vi "Read Controllers.vi"   [LabVIEW 2014]
uses:
  Begin/Global RefNums.vi
  <vilib>/Rock Robotics/WPI/Joystick/WPI_JoystickGetSetRefNum.vi
  Begin/Global Variables.vi
  <vilib>/Rock Robotics/Network Tables/SD Write Number.vi
types:
  T1 = typedef "WPI_JoystickDevRef.ctl" = cluster{"Device":T2}
  T2 = typedef "WPI_JoystickDeviceEnum.ctl" = enum16{"USB 0", "USB 1", "USB 2", "USB 3", "USB 4", "USB 5"}
  T3 = cluster{"Axes[0]":dbl, "Axes[1]":dbl, "Axes[2]":dbl, "Axes[3]":dbl, "Axes[4]":dbl, "Axes[5]":dbl, "Axes[6]":dbl, "Axes[7]":dbl, "Axes[8]":dbl}
  T4 = cluster{"Buttons[0]":bool, "Buttons[1]":bool, "Buttons[2]":bool, "Buttons[3]":bool, "Buttons[4]":bool, "Buttons[5]":bool, "Buttons[6]":bool, "Buttons[7]":bool, "Buttons[8]":bool}
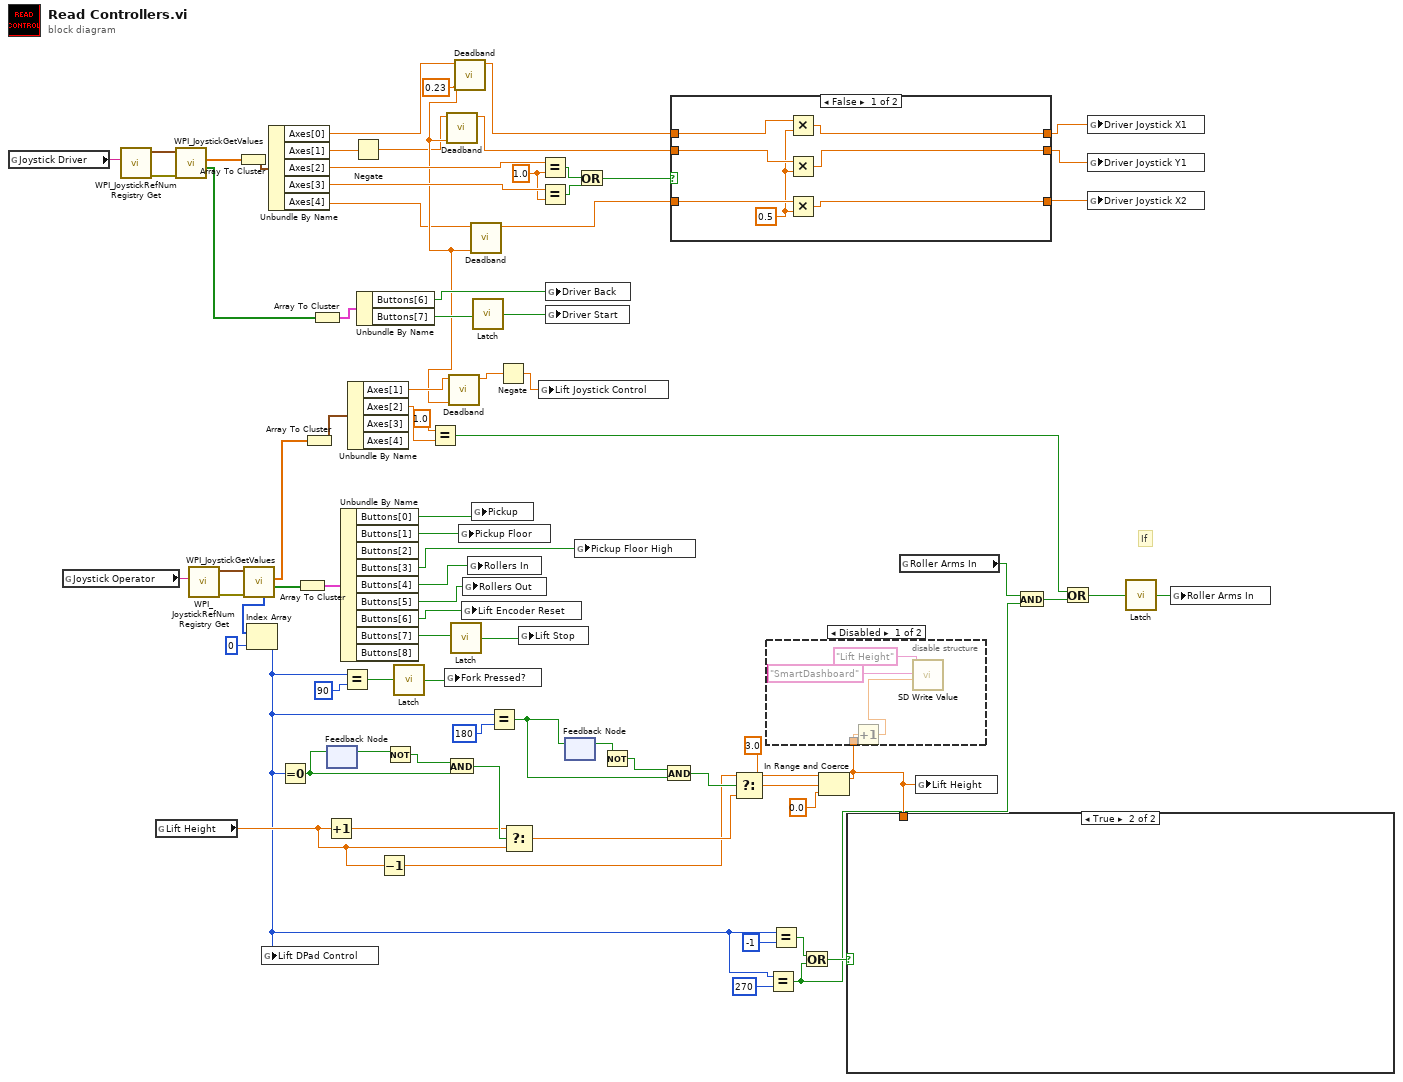
[diagram p0: block diagram]
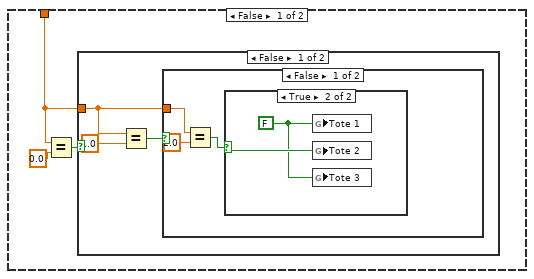
[diagram p2: hidden frame]
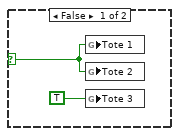
[diagram p3: hidden frame]
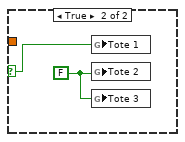
[diagram p4: hidden frame]
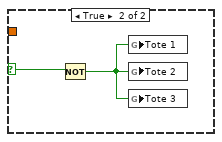
[diagram p5: hidden frame]
diagram:
  w22 = 0.23 ("Value to Deadband (default of 0.1)")
  w64 = 1.0 ("y")
  # "If"
  n1 = global read "Global RefNums.vi" "Joystick Driver"() -> (w80:string)
  n2 = global read "Global RefNums.vi" "Joystick Operator"() -> (w75:string)
  n3 = call <vilib>:"WPI_JoystickRefNum Registry Get.vi"("refnum name"=w80) -> ("error out"=w78:errorcluster, "JoystickDevRef"=w79:T1)  [unwired: 9 in]
  n4 = global read "Global Variables.vi" "Lift Height"() -> (w38:dbl)
  n5 = call <vilib>:"WPI_JoystickGetValues.vi"("error in (no error)"=w78, "JoystickDevRef"=w79) -> ("Buttons"=w63:bool[], "Axes"=w74:dbl[])  [unwired: 5 in, 3 out]
  n6 = call <vilib>:"WPI_JoystickRefNum Registry Get.vi"("refnum name"=w75) -> ("error out"=w77:errorcluster, "JoystickDevRef"=w76:T1)  [unwired: 9 in]
  n7 = Array To Cluster(array=w74) -> (cluster=w73:T3)
  n8 = call <vilib>:"WPI_JoystickGetValues.vi"("error in (no error)"=w77, "JoystickDevRef"=w76) -> ("Buttons"=w57:bool[], "Axes"=w29:dbl[], "POVs"=w51:i16[])  [unwired: 5 in, 2 out]
  n9 = Index Array(array=w51, index=0) -> (element=w11:i16)
  n10 = global write "Global Variables.vi" "Lift DPad Control"(w11) -> ()
  n11 = Unbundle By Name(w73) -> ("Axes[0]"=w58:dbl, "Axes[1]"=w13:dbl, "Axes[2]"=w69:dbl, "Axes[3]"=w65:dbl, "Axes[4]"=w14:dbl)
  n12 = Equal To 0?(x=w11) -> (x = 0?=w47:bool)
  n13 = Array To Cluster(array=w57) -> (cluster=w56:T4)
  n14 = Array To Cluster(array=w29) -> (cluster=w28:T3)
  n15 = Array To Cluster(array=w63) -> (cluster=w62:T4)
  n16 = Increment(x=w38) -> (x+1=w45:dbl)
  n17 = feedback-in #1(w47) -> ()
  n18 = feedback #1() -> (w49:bool)  [unwired: 1 in]
  n19 = Unbundle By Name(w56) -> ("Buttons[0]"=w55:bool, "Buttons[1]"=w54:bool, "Buttons[3]"=w15:bool, "Buttons[4]"=w26:bool, "Buttons[5]"=w25:bool, "Buttons[6]"=w24:bool, "Buttons[7]"=w53:bool)  [unwired: 2 out]
  n20 = Equal?(x=w11, y=i16 90) -> (x = y?=w9:bool)
  n21 = Unbundle By Name(w28) -> ("Axes[1]"=w23:dbl, "Axes[2]"=w16:dbl)  [unwired: 2 out]
  n22 = Negate(x=w13) -> (-x=w12:dbl)
  n23 = Unbundle By Name(w62) -> ("Buttons[6]"=w31:bool, "Buttons[7]"=w33:bool)
  n24 = Decrement(x=w38) -> (x-1=w37:dbl)
  n25 = Not(x=w49) -> (.not. x?=w48:bool)
  n26 = call "Latch.vi"("Input"=w9) -> ("Output"=w8:bool)
  n27 = Equal?(x=1.0, y=w16) -> (x = y?=w4:bool)
  n28 = global write "Global Variables.vi" "Fork Pressed?"(w8) -> ()
  n29 = call "Deadband.vi"("Value to Deadband (default of 0.1)"=w22, "Value"=w12) -> ("Deadbanded Value"=w60:dbl)  [unwired: 9 in]
  n30 = And(x=w48, y=w47) -> (x .and. y?=w46:bool)
  n31 = call "Deadband.vi"("Value to Deadband (default of 0.1)"=w22, "Value"=w23) -> ("Deadbanded Value"=w20:dbl)  [unwired: 9 in]
  n32 = call "Latch.vi"("Input"=w53) -> ("Output"=w52:bool)
  n33 = call "Deadband.vi"("Value to Deadband (default of 0.1)"=w22, "Value"=w58) -> ("Deadbanded Value"=w61:dbl)  [unwired: 9 in]
  n34 = global write "Global Variables.vi" "Pickup Floor"(w54) -> ()
  n35 = global write "Global Variables.vi" "Lift Encoder Reset"(w24) -> ()
  n36 = global write "Global Variables.vi" "Rollers Out"(w25) -> ()
  n37 = global write "Global Variables.vi" "Rollers In"(w26) -> ()
  n38 = call "Deadband.vi"("Value to Deadband (default of 0.1)"=w22, "Value"=w14) -> ("Deadbanded Value"=w59:dbl)  [unwired: 9 in]
  n39 = global write "Global Variables.vi" "Pickup"(w55) -> ()
  n40 = call "Latch.vi"("Input"=w33) -> ("Output"=w32:bool)
  n41 = Equal?(x=w11, y=i16 180) -> (x = y?=w43:bool)
  n42 = Negate(x=w20) -> (-x=w19:dbl)
  n43 = Select(t=w45, s=w46, f=w38) -> (s? t:f=w39:dbl)
  n44 = global write "Global Variables.vi" "Lift Stop"(w52) -> ()
  n45 = global write "Global Variables.vi" "Lift Joystick Control"(w19) -> ()
  n46 = Equal?(x=w69, y=w64) -> (x = y?=w67:bool)
  n47 = Equal?(x=w65, y=w64) -> (x = y?=w66:bool)
  n48 = global write "Global Variables.vi" "Driver Back"(w31) -> ()
  n49 = global write "Global Variables.vi" "Driver Start"(w32) -> ()
  n50 = feedback #2() -> (w42:bool)  [unwired: 1 in]
  n51 = feedback-in #2(w43) -> ()
  n52 = global write "Global Variables.vi" "Pickup Floor High"(w15) -> ()
  n53 = Or(x=w67, y=w66) -> (x .or. y?=w68:bool)
  n54 = Not(x=w42) -> (.not. x?=w41:bool)
  n55 = And(x=w41, y=w43) -> (x .and. y?=w40:bool)
  n56 = case shown="False" w68 {
    tunnel: w61 -> [w87 w88]
    tunnel: w60 -> [w86 w89]
    tunnel: w59 -> [w85 w90]
    tunnel: [w81 w90] -> w71
    tunnel: [w82 w89] -> w70
    tunnel: [w83 w88] -> w72
    frame False {
      w84 = 0.5 ("y")
      n57 = Multiply(x=w87, y=w84) -> (x*y=w83:dbl)
      n58 = Multiply(x=w86, y=w84) -> (x*y=w82:dbl)
      n59 = Multiply(x=w85, y=w84) -> (x*y=w81:dbl)
    }
    frame True {
    }
  }
  n60 = Select(t=w37, s=w40, f=w39) -> (s? t:f=w34:dbl)
  n61 = Equal?(x=w11, y=i16 270) -> (x = y?=w5:bool)
  n62 = Equal?(x=w11, y=i16 -1) -> (x = y?=w18:bool)
  n63 = Or(x=w18, y=w5) -> (x .or. y?=w7:bool)
  n64 = In Range and Coerce(upper limit=3.0, x=w34, lower limit=0.0) -> (coerced(x)=w30:dbl)  [unwired: 1 out]
  n65 = disable-structure shown="Disabled" {
    disable-tunnel: w30 -> [w92 _]
    frame Disabled {
      n66 = Increment(x=w92) -> (x+1=w91:dbl)
      n67 = call-poly <vilib>:"SD Write Value.vi"("Numeric"=w91, "Table Prefix"="SmartDashboard", "Name"="Lift Height") -> ()  [unwired: 7 in, 2 out]
    }
    frame Enabled {
    }
  }
  n68 = case shown="True" w7 {
    tunnel: w30 -> [w97 _]
    frame False {
      n69 = Equal?(x=w97, y=0.0) -> (x = y?=w96:bool)
      n70 = case shown="False" w96 {
        selector: w96 -> [_ w111]
        tunnel: w97 -> [w98 _]
        frame False {
          n71 = Equal?(x=w98, y=1.0) -> (x = y?=w99:bool)
          n72 = case shown="False" w99 {
            selector: w99 -> [_ w108]
            tunnel: w98 -> [w103 _]
            frame False {
              n73 = Equal?(x=w103, y=2.0) -> (x = y?=w101:bool)
              n74 = case shown="True" w101 {
                selector: w101 -> [w104 w107]
                frame False {
                  n75 = global write "Global Variables.vi" "Tote 1"(w104) -> ()
                  n76 = global write "Global Variables.vi" "Tote 2"(w104) -> ()
                  n77 = global write "Global Variables.vi" "Tote 3"(TRUE ("Tote 2")) -> ()
                }
                frame True {
                  w106 = FALSE ("Tote 0")
                  n78 = global write "Global Variables.vi" "Tote 1"(w106) -> ()
                  n79 = global write "Global Variables.vi" "Tote 2"(w107) -> ()
                  n80 = global write "Global Variables.vi" "Tote 3"(w106) -> ()
                }
              }
            }
            frame True {
              w109 = FALSE ("Tote 1")
              n81 = global write "Global Variables.vi" "Tote 1"(w108) -> ()
              n82 = global write "Global Variables.vi" "Tote 2"(w109) -> ()
              n83 = global write "Global Variables.vi" "Tote 3"(w109) -> ()
            }
          }
        }
        frame True {
          n84 = Not(x=w111) -> (.not. x?=w110:bool)
          n85 = global write "Global Variables.vi" "Tote 1"(w110) -> ()
          n86 = global write "Global Variables.vi" "Tote 2"(w110) -> ()
          n87 = global write "Global Variables.vi" "Tote 3"(w110) -> ()
        }
      }
    }
    frame True {
    }
  }
  n88 = global read "Global Variables.vi" "Roller Arms In"() -> (w6:bool)
  n89 = global write "Global Variables.vi" "Lift Height"(w30) -> ()
  n90 = And(x=w6, y=w5) -> (x .and. y?=w3:bool)
  n91 = Or(x=w4, y=w3) -> (x .or. y?=w2:bool)
  n92 = global write "Global Variables.vi" "Driver Joystick X1"(w72) -> ()
  n93 = global write "Global Variables.vi" "Driver Joystick Y1"(w70) -> ()
  n94 = global write "Global Variables.vi" "Driver Joystick X2"(w71) -> ()
  n95 = call "Latch.vi"("Input"=w2) -> ("Output"=w1:bool)
  n96 = global write "Global Variables.vi" "Roller Arms In"(w1) -> ()
